vi "Tools_String RFC-1123 Date.vi"(0 "time (now)":dbl format="%.2f", 1 "numeric zone offset (true)":bool=TRUE) -> (2 "GMT Date/Time":string)   [LabVIEW 2017]
doc: "Formats time according to RFC-1123.\n\ntime - time to be formated (defaults to current time)\n\nnumeric zone offset -\n if TRUE, formats to local time with GMT offset\n if FALSE, formats to GMT time"
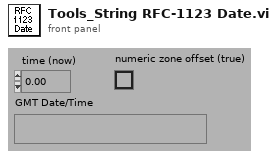
[diagram p1: front panel]
types:
  T1 = cluster{"second":i32, "minute":i32, "hour":i32, "day of month":i32, "month":i32, "year":i32, "day of week":i32, "day of year":i32, "is DST":i32}
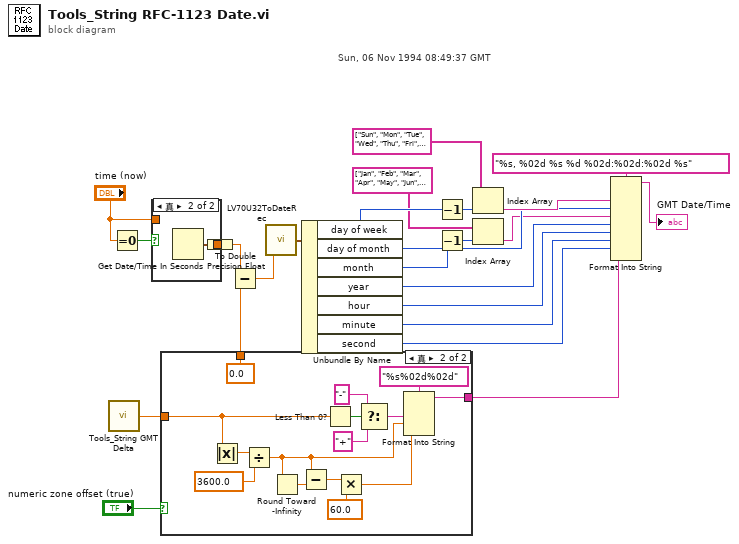
[diagram p0: block diagram]
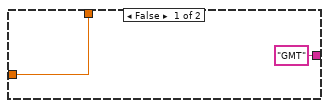
[diagram p2: hidden frame]
diagram:
  # "Sun, 06 Nov 1994 08:49:37 GMT"
  n1 = call "Tools_String GMT Delta.vi"() -> ("GMT Delta in seconds"=w2:dbl)
  n2 = Equal To 0?(x="time (now)") -> (x = 0?=w6:bool)
  n3 = case shown="真" w6 {
    tunnel: [w25 w27] -> w8
    tunnel: "time (now)" -> [w25 _]
    frame False {
    }
    frame True {
      n4 = Get Date/Time In Seconds() -> (seconds since 1Jan1904=w26:timestamp)
      n5 = To Double Precision Float(number=w26) -> (double precision float=w27:dbl)
    }
  }
  n6 = case shown="真" "numeric zone offset (true)" {
    tunnel: ["GMT" w41] -> w4
    tunnel: w2 -> [w28 w39]
    tunnel: [w28 0.0 ("GMT Delta in seconds")] -> w1
    frame False {
    }
    frame True {
      n7 = Absolute Value(x=w39) -> (abs(x)=w38:dbl)
      n8 = Divide(x=w38, y=3600.0) -> (x/y=w42:dbl)
      n9 = Round Toward -Infinity(1:w42) -> (0:w35:dbl)
      n10 = Subtract(x=w42, y=w35) -> (x-y=w36:dbl)
      n11 = Less Than 0?(x=w39) -> (x < 0?=w32:bool)
      n12 = Multiply(x=w36, y=60.0) -> (x*y=w43:dbl)
      n13 = Select(t="-", s=w32, f="+") -> (s? t:f=w44:string)
      n14 = Format Into String(format string="%s%02d%02d", w44, w42, w43) -> (resulting string=w41:string)  [unwired: 2 in, 1 out]
    }
  }
  n15 = Subtract(x=w8, y=w1) -> (x-y=w7:dbl)
  n16 = call <vilib>:"LV70U32ToDateRec.vi"("Time"=w7) -> ("date time rec"=w20:T1)
  n17 = Unbundle By Name(w20) -> ("day of week"=w19:i32, "day of month"=w18:i32, "month"=w10:i32, "year"=w17:i32, "hour"=w16:i32, "minute"=w15:i32, "second"=w14:i32)
  n18 = Decrement(x=w19) -> (x-1=w22:i32)
  n19 = Decrement(x=w10) -> (x-1=w11:i32)
  n20 = Index Array(array=string[] ["Sun", "Mon", "Tue", "Wed", "Thu", "Fri", "Sat"], index=w22) -> (element=w21:string)
  n21 = Index Array(array=string[] ["Jan", "Feb", "Mar", "Apr", "May", "Jun", "Jul", "Aug", "Sep", "Oct", "Nov", "Dec"], index=w11) -> (element=w13:string)
  n22 = Format Into String(format string="%s, %02d %s %d %02d:%02d:%02d %s", w21, w18, w13, w17, w16, w15, w14, w4) -> (resulting string=→"GMT Date/Time":string)  [unwired: 2 in, 1 out]
